vi "Camera Pixel to Angle.vi"(9 "Split Image Info":T1={"height"=120.0, "width"=120.0, "deg/pix"=120.0}, 11 "Point (px)":cluster{"X":dbl, "Y":dbl}) -> (3 "angle":dbl)   [LabVIEW 2025]
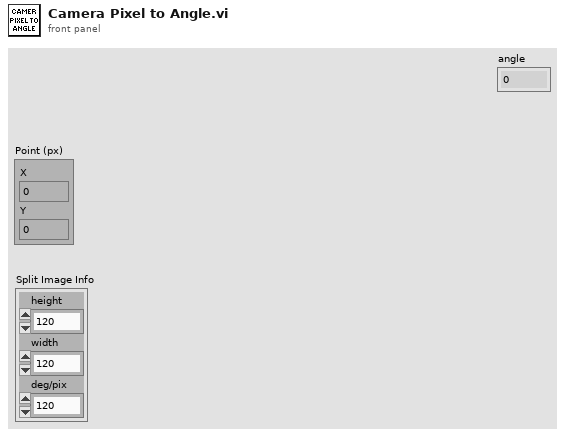
[diagram p1: front panel]
types:
  T1 = cluster{"height":dbl, "width":dbl, "deg/pix":dbl}
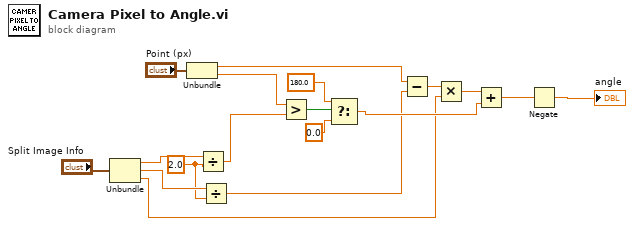
[diagram p0: block diagram]
diagram:
  w6 = 2.0 ("y")
  n1 = Unbundle("Split Image Info") -> ("height"=w7:dbl, "width"=w8:dbl, "deg/pix"=w2:dbl)
  n2 = Unbundle("Point (px)") -> ("X"=w18:dbl, "Y"=w15:dbl)
  n3 = Divide(x=w7, y=w6) -> (x/y=w5:dbl)
  n4 = Divide(x=w8, y=w6) -> (x/y=w4:dbl)
  n5 = Greater?(x=w15, y=w5) -> (0:w16:bool)
  n6 = Select(t=180.0, s=w16, f=0.0) -> (s? t:f=w11:dbl)
  n7 = Subtract(x=w18, y=w4) -> (x-y=w3:dbl)
  n8 = Multiply(x=w3, y=w2) -> (x*y=w12:dbl)
  n9 = Add(x=w12, y=w11) -> (x+y=w10:dbl)
  n10 = Negate(x=w10) -> (-x=→"angle":dbl)
